vi "RSZVB Calibration Auto Simplified.vi"(4 "Analyzer Port 1 (1)":i32=1, 5 "Analyzer Port 4 (0)":i32, 6 "Analyzer Port 3 (0)":i32, 7 "Analyzer Port 2 (0)":i32, 8 "error in (no error)":errorcluster {"code" format="%.0x"}, 9 "Calibration Kit Name":string, 10 "Channel (1)":i32=1, 11 "VISA session":refnum<visa-resource-name>) -> (0 "error out":errorcluster {"code" format="%.0x"}, 3 "dup VISA session":refnum<visa-resource-name>)   [LabVIEW 2011]
doc: "This VI selects and initiates a one-port, two-port, three-port or four-port automatic calibration at arbitrary analyzer ports.\n\nNote(s):\n\n(1) If the test setup contains a high attenuation the analyzer may fail to detect the cal unit ports connected to each of its ports. In this case use the extended VI rszvb_CalibrationAuto (command [SENSe<Ch>:]CORRection:COLLect:AUTO:PORTs)\n\n \nRemote-control command(s):\n[SENSe<Ch>:]CORRection:COLLect:AUTO '<file_name>',<port_no>{,<port_no>}"
uses:
  _utility/RSZVB Global Data.vi
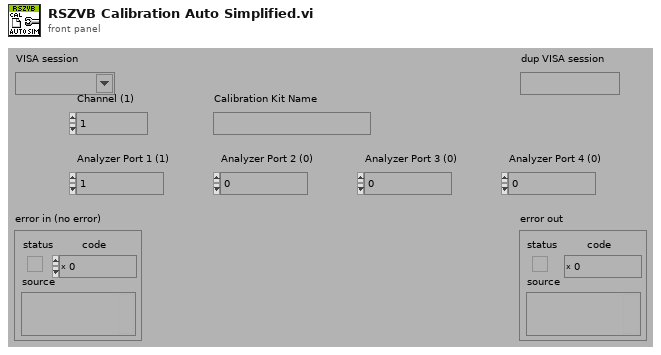
[diagram p1: front panel]
types:
  T1 = cluster{"Error Checking (T: On)":bool, "Installed Options":string[], "Data Valid?":bool, "Ports":i32, "Model":string[], "Option Checking (T: On)":bool}[]
  T2 = cluster{"Error Checking (T: On)":bool, "Installed Options":string[], "Data Valid?":bool, "Ports":i32, "Model":string[], "Option Checking (T: On)":bool}
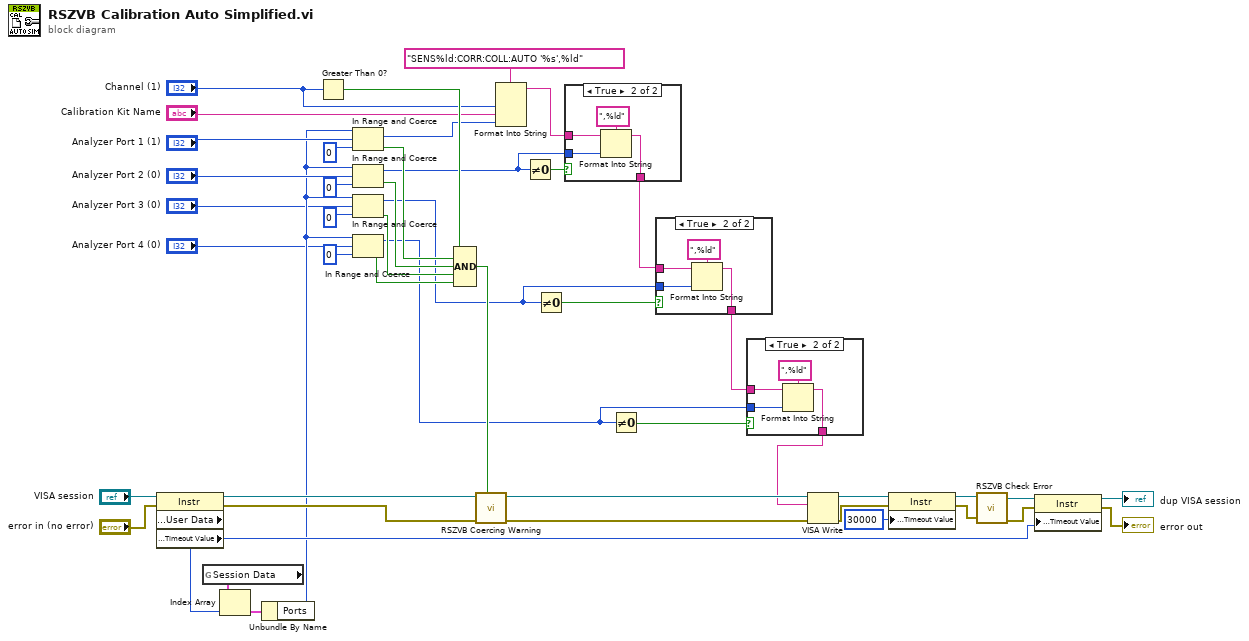
[diagram p0: block diagram]
diagram:
  n1 = property class="Instr"(reference="VISA session", error in="error in (no error)") -> (reference out=w40:refnum<visa-resource-name>, error out=w41:errorcluster, "General Settings:User Data"=w13:u32, "General Settings:Timeout Value"=w27:u32)
  n2 = global read "RSZVB Global Data.vi" "Session Data"() -> (w42:T1)
  n3 = Index Array(array=w42, index=w13) -> (element=w43:T2)
  n4 = Unbundle By Name(w43) -> ("Ports"=w14:i32)
  n5 = Greater Than 0?(x="Channel (1)") -> (x > 0?=w44:bool)
  n6 = In Range and Coerce(upper limit=w14, x="Analyzer Port 1 (1)", lower limit=0) -> (coerced(x)=w29:i32, In Range?=w36:bool)
  n7 = In Range and Coerce(upper limit=w14, x="Analyzer Port 2 (0)", lower limit=0) -> (coerced(x)=w5:i32, In Range?=w35:bool)
  n8 = In Range and Coerce(upper limit=w14, x="Analyzer Port 3 (0)", lower limit=0) -> (coerced(x)=w3:i32, In Range?=w34:bool)
  n9 = In Range and Coerce(upper limit=w14, x="Analyzer Port 4 (0)", lower limit=0) -> (coerced(x)=w4:i32, In Range?=w33:bool)
  n10 = Compound Arithmetic op=AND(w44, w36, w35, w34, w33) -> (w45:bool)
  n11 = call "RSZVB Coercing Warning.vi"("In Range?"=w45, "error in (no error)"=w41, "VISA session"=w40) -> ("error out"=w46:errorcluster, "dup VISA session"=w47:refnum<visa-resource-name>)  [unwired: 7 in]
  n12 = Format Into String(format string="SENS%ld:CORR:COLL:AUTO '%s',%ld", "Channel (1)", "Calibration Kit Name", w29) -> (resulting string=w30:string)  [unwired: 2 in, 1 out]
  n13 = Not Equal To 0?(x=w5) -> (x != 0?=w31:bool)
  n14 = Not Equal To 0?(x=w3) -> (x != 0?=w12:bool)
  n15 = case shown="True" w31 {
    tunnel: w30 -> [w49 w53]
    tunnel: w5 -> [_ w51]
    tunnel: [w49 w50] -> w8
    frame False {
    }
    frame True {
      n16 = Format Into String(format string=",%ld", initial string=w53, w51) -> (resulting string=w50:string)  [unwired: 1 in, 1 out]
    }
  }
  n17 = Not Equal To 0?(x=w4) -> (x != 0?=w11:bool)
  n18 = case shown="True" w12 {
    tunnel: w8 -> [w54 w58]
    tunnel: w3 -> [_ w56]
    tunnel: [w54 w55] -> w7
    frame False {
    }
    frame True {
      n19 = Format Into String(format string=",%ld", initial string=w58, w56) -> (resulting string=w55:string)  [unwired: 1 in, 1 out]
    }
  }
  n20 = case shown="True" w11 {
    tunnel: w7 -> [w59 w63]
    tunnel: w4 -> [_ w61]
    tunnel: [w59 w60] -> w6
    frame False {
    }
    frame True {
      n21 = Format Into String(format string=",%ld", initial string=w63, w61) -> (resulting string=w60:string)  [unwired: 1 in, 1 out]
    }
  }
  n22 = VISA Write(VISA resource name=w47, write buffer=w6, error in (no error)=w46) -> (VISA resource name out=w23:refnum<visa-resource-name>, error out=w22:errorcluster)  [unwired: 1 out]
  n23 = property class="Instr"(reference=w23, error in=w22, "General Settings:Timeout Value"=u32 30000) -> (reference out=w24:refnum<visa-resource-name>, error out=w21:errorcluster)
  n24 = call "RSZVB Check Error.vi"("error in (no error)"=w21, "VISA session"=w24) -> ("error out"=w26:errorcluster, "dup VISA session"=w25:refnum<visa-resource-name>)  [unwired: 8 in]
  n25 = property class="Instr"(reference=w25, error in=w26, "General Settings:Timeout Value"=w27) -> (reference out=→"dup VISA session":refnum<visa-resource-name>, error out=→"error out":errorcluster)
